vi "QCP_Get_I32.vi"(0 "QCP Data Block In":T1, 1 "QCP Name":string, 3 "Error In":errorcluster) -> (7 "QCP Data Block Out":T1, 9 "Value Out":i32=2147483647, 10 "Error Out":errorcluster)   [LabVIEW 2015]
uses:
  <userlib>/836-Library/System/QCP_Support_Code/QCP_Data_Block.ctl
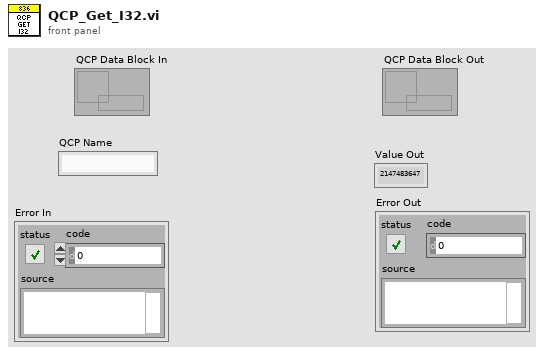
[diagram p1: front panel]
types:
  T1 = typedef "QCP_Data_Block.ctl" = refnum<data-value>
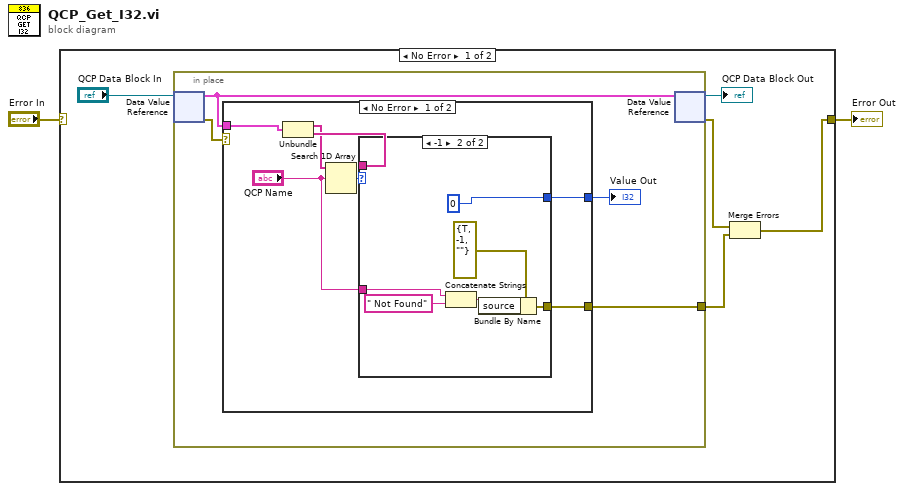
[diagram p0: block diagram]
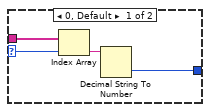
[diagram p2: hidden frame]
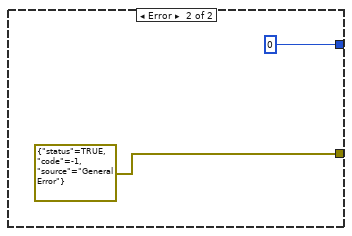
[diagram p3: hidden frame]
diagram:
  n1 = case shown="No Error" "Error In" {
    selector: "Error In" -> [_ w31]
    tunnel: [w3 w31] -> w1
    frame No Error {
      n2 = in-place {
        in-place-border: [w8] -> w4
        n3 = in-place-dvr #1("QCP Data Block In") -> (w10:cluster{string[], string[]}, w11:errorcluster)
        n4 = case shown="No Error" w11 {
          tunnel: w10 -> [w15 _]
          tunnel: [w14 0] -> w9
          tunnel: [w12 errorcluster {"status"=TRUE, "code"=-1, "source"="General Error"} ("error constant")] -> w8
          frame No Error {
            n5 = Unbundle(w15) -> (w17:string[], w18:string[])
            n6 = Search 1D Array(1D array=w17, element="QCP Name") -> (index of element=w16:i32)  [unwired: 1 out]
            n7 = case shown="-1" w16 {
              selector: w16 -> [w22 _]
              tunnel: [w19 0] -> w14
              tunnel: w18 -> [w21 _]
              tunnel: "QCP Name" -> [_ w24]
              tunnel: [_ w23] -> w12
              frame 0, Default {
                n8 = Index Array(array=w21, index=w22) -> (element=w20:string)
                n9 = Decimal String To Number(string=w20) -> (number=w19:i32)  [unwired: 2 in, 1 out]
              }
              frame -1 {
                n10 = Concatenate Strings(w24, " Not Found") -> (w25:string)
                n11 = Bundle By Name(cluster=errorcluster {"status"=TRUE, "code"=-1, "source"=""} ("error constant"), "source"=w25) -> (w23:errorcluster)
              }
            }
          }
          frame Error {
          }
        }
        "Value Out" <- w9
        n12 = in-place-dvr #1(w10) -> (→"QCP Data Block Out":T1, w5:errorcluster)
      }
      n13 = Merge Errors(w5, w4) -> (w3:errorcluster)
    }
    frame Error {
    }
  }
  "Error Out" <- w1
